vi "Exemple_Preprocessing_power_transform.vi"() -> ()   [LabVIEW 2020]
panel:
  out "Data":T1
  out "error out":errorcluster
  in  "X":string[][](array[string])=[["1", "2"], ["3", "2"], ["4", "5"]]
  in  "error in":errorcluster caption="entrée d'erreur"
  in  "power_transform":T2={"method"="box-cox", "standardize"=TRUE, "copy"=TRUE}
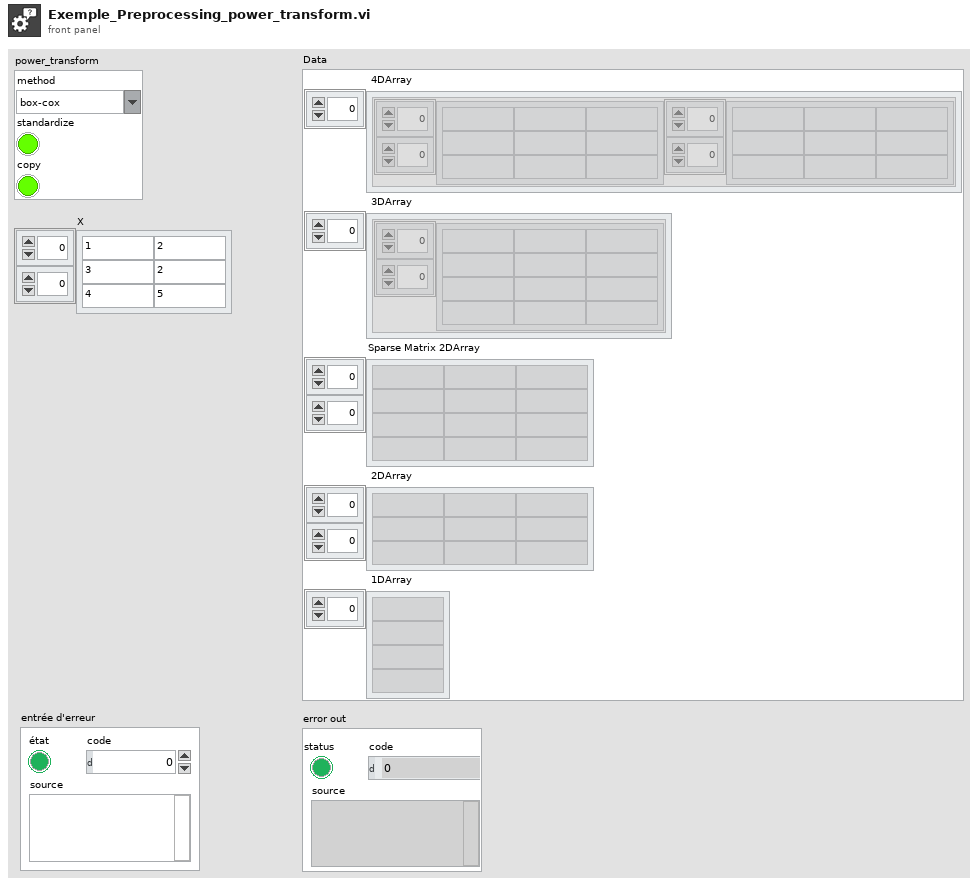
[diagram p1: front panel]
types:
  T1 = cluster{" 4DArray":cluster{"1":string[][], "2":string[][]}[], " 3DArray":cluster{"Tableau":string[][]}[], "Sparse Matrix 2DArray":string[][], " 2DArray":string[][], " 1DArray":string[]}
  T2 = cluster{"method":string, "standardize":bool, "copy":bool}
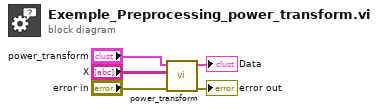
[diagram p0: block diagram]
diagram:
  n1 = call "power_transform.vi"("error in"="error in", "X"="X", "power_transform"="power_transform") -> ("error out"=→"error out":errorcluster, "Data"=→"Data":T1)  [unwired: 7 in]
